vi "AIK.vi"(8 "error in (no error)":errorcluster, 10 "p":dbl[](array[numeric]), 11 "Delta Robot Kinematics in":refnum<class "Delta Robot Kinematics.lvclass">) -> (0 "error out":errorcluster, 1 "exist":bool, 2 "joints":dbl[](array[numeric]), 3 "Delta Robot Kinematics out":refnum<class "Delta Robot Kinematics.lvclass">)   [LabVIEW 2013, in "Delta Robot Kinematics.lvclass"]
uses:
  Delta Robot Kinematics.lvclass
  Delta Robot Kinematics.lvclass/Delta Robot Kinematics.ctl
  <vilib>/Analysis/baseanly.llb/A x Vector.vi
  <vilib>/Analysis/_algsub.llb/Vector Norm.vi
  <vilib>/Analysis/_algsub.llb/Real Vector Norm.vi
  <vilib>/Analysis/baseanly.llb/Outer Product.vi
  <vilib>/Analysis/baseanly.llb/Real Outer Product.vi
  <vilib>/robotics/Kinematics/Create Lie Group Matrix.vi
  <vilib>/Analysis/7linalg.llb/Create Special Matrix.vi
  <vilib>/Analysis/7linalg.llb/Create Special Real Matrix.vi
  <vilib>/Analysis/Matrix/Numeric/Multiply/Multiply.vi
  <vilib>/Analysis/Matrix/Numeric/Multiply/Multiply - RM,R.vi
  <vilib>/Analysis/Matrix/Numeric/Multiply/Multiply - R,RM.vi
  <vilib>/Analysis/Matrix/Numeric/Add/Add.vi
  <vilib>/Analysis/Matrix/Numeric/Add/Add - RM,RM.vi
  <vilib>/robotics/Kinematics/NI_Kinematics.lvlib
  <vilib>/Analysis/NI_AALBase.lvlib
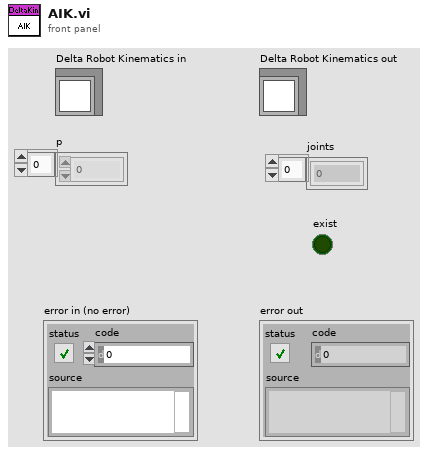
[diagram p1: front panel]
types:
  T1 = typedef "NI_Matrix.lvlib/RealMatrix.ctl" = dbl[][]
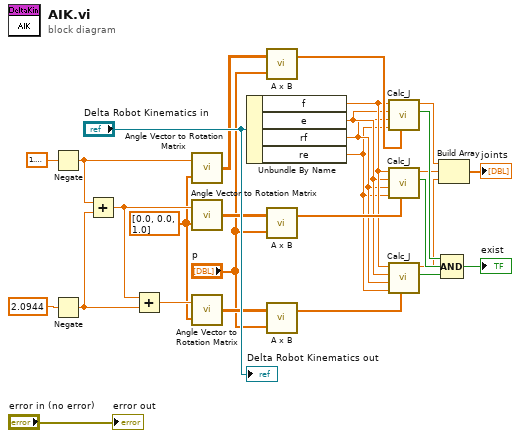
[diagram p0: block diagram]
diagram:
  w21 = dbl[] [0.0, 0.0, 1.0] ("vector")
  n1 = Negate(x=1.5707963267948966) -> (-x=w25:dbl)
  n2 = Negate(x=2.0944 ("y")) -> (-x=w9:dbl)
  n3 = Add(x=w25, y=w9) -> (x+y=w22:dbl)
  n4 = Add(x=w22, y=w9) -> (x+y=w23:dbl)
  n5 = call <vilib>:"Angle Vector to Rotation Matrix.vi"("vector"=w21, "angle"=w25) -> ("rotation matrix"=w11:T1)
  n6 = call <vilib>:"Angle Vector to Rotation Matrix.vi"("vector"=w21, "angle"=w22) -> ("rotation matrix"=w24:T1)
  n7 = call <vilib>:"Angle Vector to Rotation Matrix.vi"("vector"=w21, "angle"=w23) -> ("rotation matrix"=w20:T1)
  n8 = Unbundle By Name("Delta Robot Kinematics in") -> ("f"=w6:dbl, "e"=w5:dbl, "rf"=w4:dbl, "re"=w3:dbl)
  n9 = call-poly <vilib>:"A x B.vi"("Vector"="p", "A"=w11) -> ("A x Vector"=w26:dbl[])  [unwired: 1 out]
  n10 = call-poly <vilib>:"A x B.vi"("Vector"="p", "A"=w24) -> ("A x Vector"=w19:dbl[])  [unwired: 1 out]
  n11 = call-poly <vilib>:"A x B.vi"("Vector"="p", "A"=w20) -> ("A x Vector"=w18:dbl[])  [unwired: 1 out]
  n12 = call "Calc_J.vi"("p"=w26, "re"=w3, "rf"=w4, "e"=w5, "f"=w6) -> ("exist"=w17:bool, "theta"=w14:dbl)  [unwired: 5 in]
  n13 = call "Calc_J.vi"("p"=w19, "re"=w3, "rf"=w4, "e"=w5, "f"=w6) -> ("exist"=w16:bool, "theta"=w13:dbl)  [unwired: 5 in]
  n14 = call "Calc_J.vi"("p"=w18, "re"=w3, "rf"=w4, "e"=w5, "f"=w6) -> ("exist"=w15:bool, "theta"=w12:dbl)  [unwired: 5 in]
  n15 = Build Array(w14, w13, w12) -> (→"joints":dbl[])
  n16 = Compound Arithmetic op=AND(w17, w16, w15) -> (→"exist":bool)
  "Delta Robot Kinematics out" <- "Delta Robot Kinematics in"
  "error out" <- "error in (no error)"
